vi "Set Prev Action.vi"(7 "Action":T1, 8 "error in (no error)":errorcluster, 10 "Payload":variant, 11 "queue in":refnum<queue>) -> (0 "error out":errorcluster, 3 "queue out":refnum<queue>)   [LabVIEW 2010]
uses:
  RF Characterization States.ctl
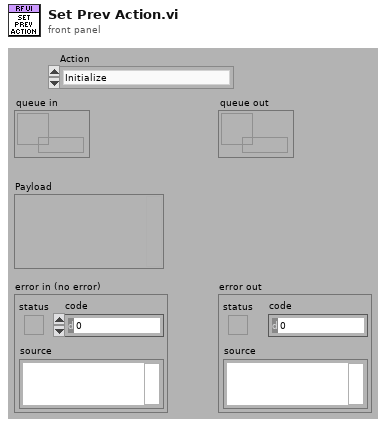
[diagram p1: front panel]
types:
  T1 = typedef "RF Characterization States.ctl" = enum16{"Initialize", "Enable/Disable Navigation", "Set Next Action", "Set Prev Action", "Set Stop Action", "Prev Action Triggered", "Next Action Triggered", "Stop Action Triggered", "Move Gantry to Position", "Display Configuration Tab", "Check Configuration", "Display Attenuation Tab", "Check Attenuation Config", "Start Attenuation Test", "Check Attenuation Results", "Display Power Tab", "Check Power Config", "Start Power Test", "Check Power Results", "Display Mapping Tab", "Check Mapping Config", "Start Mapping Test", "Take Mapping Sample", "Finish Mapping Test", "Check Mapping Results", "Display Report Tab", "Generate Report", "Save Report", "Error", "Shutdown"}
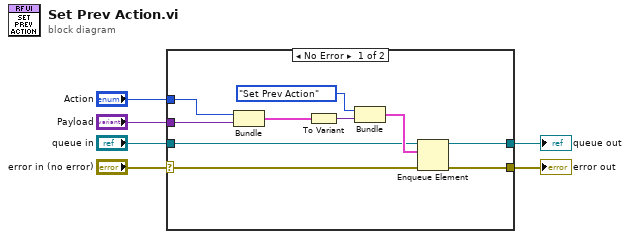
[diagram p0: block diagram]
diagram:
  n1 = case shown="No Error" "error in (no error)" {
    selector: "error in (no error)" -> [w7 w17]
    tunnel: [w16 w17] -> w6
    tunnel: [w15 w18] -> w5
    tunnel: "queue in" -> [w13 w18]
    tunnel: "Payload" -> [w11 _]
    tunnel: "Action" -> [w10 _]
    frame No Error {
      n2 = Bundle("Action"=w10, "Payload"=w11) -> (w9:cluster{"Action":T1, "Payload":variant})  [unwired: 1 in]
      n3 = To Variant(anything=w9) -> (Variant=w8:variant)
      n4 = Bundle("State"=RF_Characterization_States."Set Prev Action", "Variant"=w8) -> (w14:cluster{"State":T1, "Variant":variant})  [unwired: 1 in]
      n5 = Enqueue Element(queue=w13, element=w14, error in (no error)=w7) -> (queue out=w15:refnum<queue>, error out=w16:errorcluster)  [unwired: 1 in, 1 out]
    }
    frame Error {
    }
  }
  "error out" <- w6
  "queue out" <- w5
